vi "PwF_ToF_GetDistance.vi"(0 "PwF ToF Ref":T1, 11 "error in (no error)":errorcluster) -> (4 "PwF ToF Ref":T1, 6 "Dist_mm":u16, 8 "RangingStatus":u8, 10 "MeasQuality":u8, 14 "SigRetRate":dbl, 15 "error out":errorcluster)   [LabVIEW 2018]
uses:
  ToF_TypeDef/PwF ToF Ref.ctl
  ToF_TypeDef/PwF ToF RangingMode.ctl
panel:
  out "Message ID Out":u32 format="%.0x"
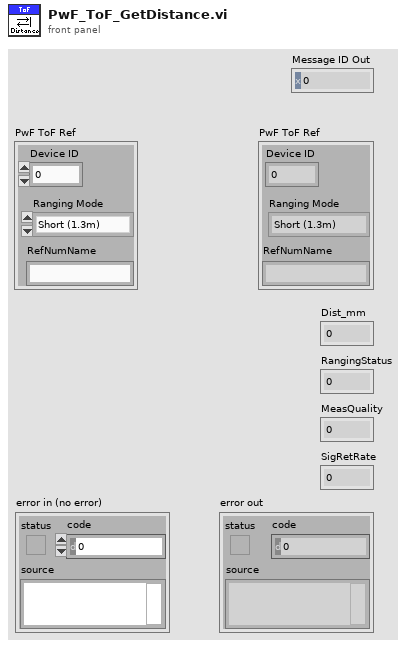
[diagram p1: front panel]
types:
  T1 = typedef "PwF ToF Ref.ctl" = cluster{"Device ID":u8, "Ranging Mode":T2, "RefNumName":string}
  T2 = typedef "PwF ToF RangingMode.ctl" = enum8{"Short (1.3m)", "Medium (2m)", "Long (4m)"}
  T3 = cluster{"Data[0]":u8, "Data[1]":u8, "Data[2]":u8, "Data[3]":u8, "Data[4]":u8, "Data[5]":u8, "Data[6]":u8, "Data[7]":u8, "Data[8]":u8}
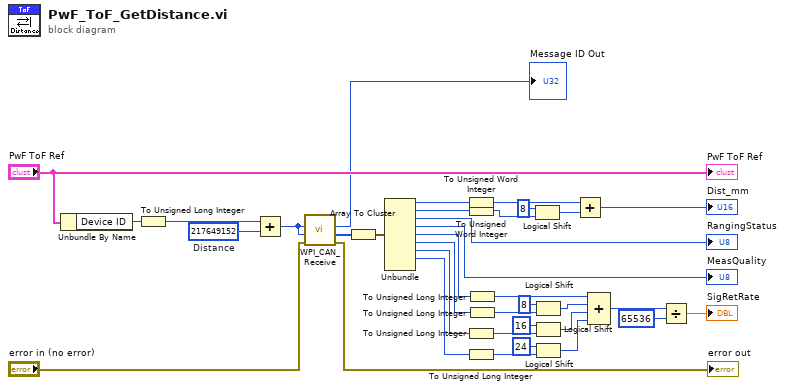
[diagram p0: block diagram]
diagram:
  w35 = u32 217649152  # Distance
  n1 = Unbundle By Name("PwF ToF Ref") -> ("Device ID"=w36:u8)
  n2 = To Unsigned Long Integer(number=w36) -> (unsigned 32bit integer=w2:u32)
  n3 = Add(x=w2, y=w35) -> (x+y=w34:u32)
  n4 = call <vilib>:"WPI_CAN_Receive.vi"("error in (no error)"="error in (no error)", "Message ID Mask"=w34, "Message ID"=w34) -> ("error out"=→"error out":errorcluster, "Data"=w23:u8[], "Message ID Out"=→"Message ID Out":u32)  [unwired: 6 in]
  n5 = Array To Cluster(array=w23) -> (cluster=w18:T3)
  n6 = Unbundle(w18) -> ("Data[0]"=w17:u8, "Data[1]"=w20:u8, "Data[2]"=→"RangingStatus":u8, "Data[3]"=→"MeasQuality":u8, "Data[4]"=w11:u8, "Data[5]"=w8:u8, "Data[6]"=w9:u8, "Data[7]"=w10:u8)  [unwired: 1 out]
  n7 = To Unsigned Word Integer(number=w17) -> (unsigned 16bit integer=w16:u16)
  n8 = To Unsigned Word Integer(number=w20) -> (unsigned 16bit integer=w19:u16)
  n9 = To Unsigned Long Integer(number=w9) -> (unsigned 32bit integer=w14:u32)
  n10 = To Unsigned Long Integer(number=w10) -> (unsigned 32bit integer=w15:u32)
  n11 = To Unsigned Long Integer(number=w11) -> (unsigned 32bit integer=w12:u32)
  n12 = To Unsigned Long Integer(number=w8) -> (unsigned 32bit integer=w13:u32)
  n13 = Logical Shift(y=i16 8, x=w19) -> (x << y=w22:u16)
  n14 = Logical Shift(y=i16 8, x=w13) -> (x << y=w29:u32)
  n15 = Logical Shift(y=i16 16, x=w14) -> (x << y=w28:u32)
  n16 = Logical Shift(y=i16 24, x=w15) -> (x << y=w27:u32)
  n17 = Add(x=w16, y=w22) -> (x+y=→"Dist_mm":u16)
  n18 = Compound Arithmetic op=ADD(w12, w29, w28, w27) -> (w24:u32)
  n19 = Divide(x=w24, y=u32 65536) -> (x/y=→"SigRetRate":dbl)
  "PwF ToF Ref" <- "PwF ToF Ref"
